vi "PXI-4132 Global Variable.vi"() -> ()   [LabVIEW 2013, in "PXI-4132 Custom Device.lvlib"]
uses:
  PXI-4132 Custom Device.lvlib
panel:
  in  "Continuous Read?":string="Continuous Read?"
  in  "Read Trigger":string="Read Trigger"
  in  "Channel #":string="Channel #"
  in  "Channel 0 Type":string="Channel 0 Type"
  in  "Channel 0 Sense":string="Channel 0 Sense"
  in  "Hardware Device Name":string="Hardware Device Name"
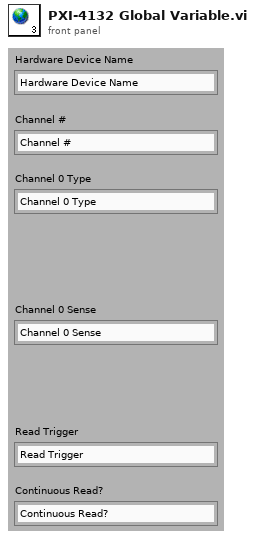
[diagram p1: front panel]
diagram:
